vi "write buffer.vi"(8 "error in (no error)":errorcluster, 10 "Data":dbl[](array[numeric]), 11 "Data Buffer in":refnum<class "Data Buffer.lvclass">) -> (0 "error out":errorcluster, 2 "XY Graph":T1(array[cluster]), 3 "Data Buffer out":refnum<class "Data Buffer.lvclass">)   [LabVIEW 2022 SP3, in "Data Buffer.lvclass"]
uses:
  Data Buffer.lvclass
  Data Buffer.lvclass/Data Buffer.ctl
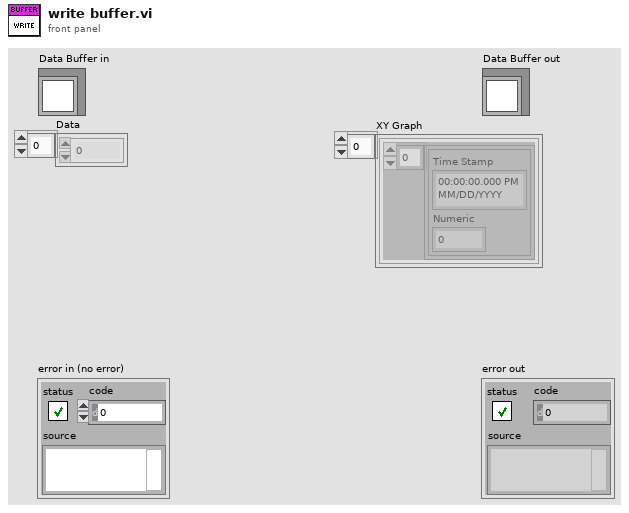
[diagram p1: front panel]
types:
  T1 = cluster{cluster{"Time Stamp":timestamp, "Numeric":dbl}[]}[]
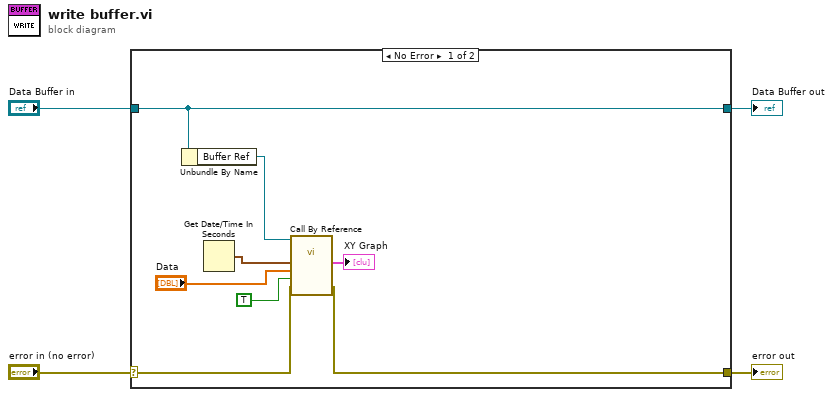
[diagram p0: block diagram]
diagram:
  n1 = case shown="No Error" "error in (no error)" {
    selector: "error in (no error)" -> [w8 w14]
    tunnel: [w7 w14] -> w3
    tunnel: [w12 w13] -> w1
    tunnel: "Data Buffer in" -> [w12 w13]
    frame No Error {
      n2 = Unbundle By Name(w12) -> ("Buffer Ref"=w11:refnum<vi>)
      n3 = Get Date/Time In Seconds() -> (seconds since 1Jan1904=w6:timestamp)
      n4 = call-by-ref "?"(reference=w11, "error in (no error)"=w8, "Write?"=TRUE, "Data"="Data", "Time Stamp"=w6) -> ("error out"=w7:errorcluster, "XY Graph"=→"XY Graph":T1)  [unwired: 7 in, 2 out]
    }
    frame Error {
    }
  }
  "error out" <- w3
  "Data Buffer out" <- w1
